vi "Toggle Debugging_Item_OnPopupMenu.vi"(11 "Object":T1) -> ()   [LabVIEW 2015]
uses:
  <resource>/Framework/Providers/API/ItemRef.ctl
  <resource>/Framework/Providers/API/mxLvMenuItem.ctl
panel:
  out "error out":errorcluster
  in  "error in":errorcluster
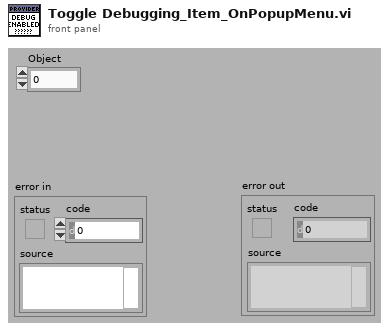
[diagram p1: front panel]
types:
  T1 = typedef "ItemRef.ctl" = u64
  T2 = typedef "mxLvMenuItem.ctl" = cluster{"Menu Name":string, "Description":string, "Icon File Name":path, "Menu Tag":string, "Enabled":bool, "Checked":bool, "Separator":bool, "Batchable":bool, "Weight":i32, "Batch Mode (Ignored if Not Batchable)":enum32{"Show If All Items Support Command", "Show If Any Items Support Command"}, "Menu Location":enum32{"<None>", "Project", "Project / Build Specifications", "Tools", "Tools / Source Control", "Tools / Real-Time Module", "Help"}, "Exclude From Getting Started Window Menu":bool}
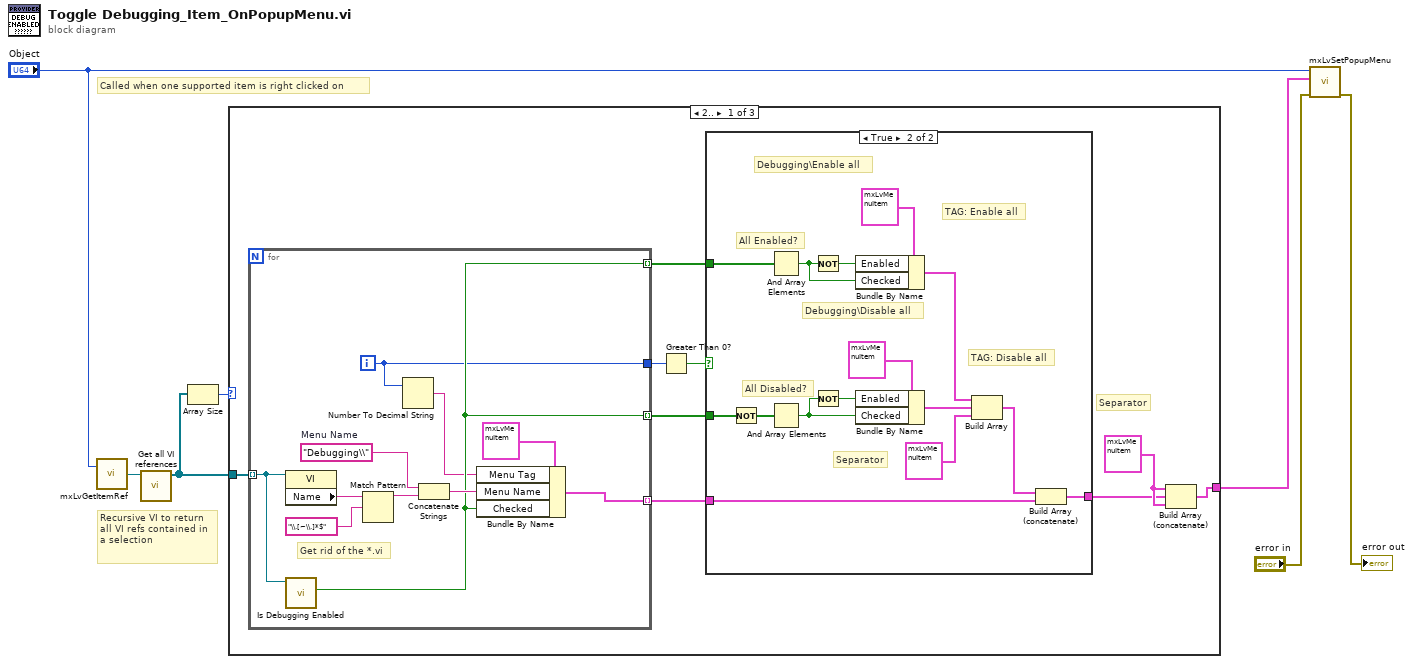
[diagram p0: block diagram]
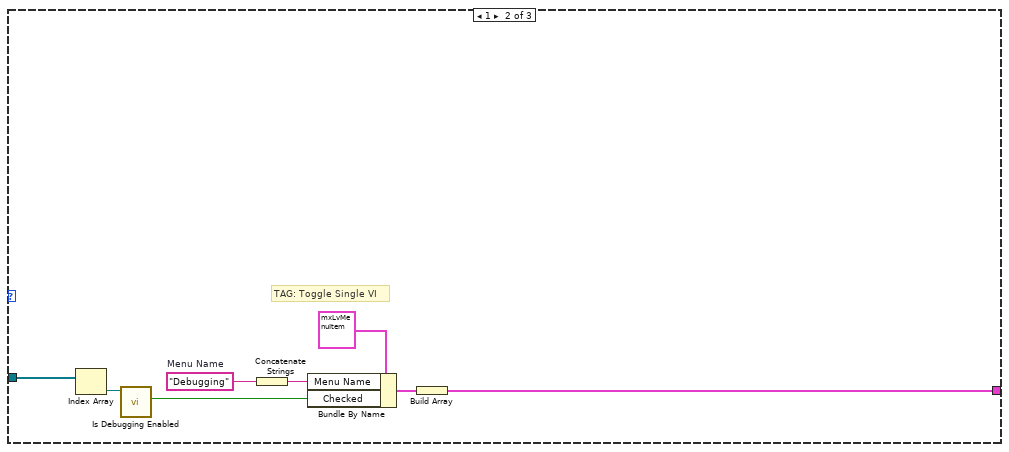
[diagram p3: hidden frame]
diagram:
  # "Recursive VI to return all VI refs contained in a selection"
  # "Called when one supported item is right clicked on"
  n1 = call <resource>:"mxLvGetItemRef.vi"("Item"="Object") -> ("Item Refnum"=w3:refnum<vi>)  [unwired: 1 in, 2 out]
  n2 = call "Get all VI references.vi"("Project Item"=w3) -> ("VI Refs"=w1:refnum<vi>[])  [unwired: 9 in, 1 out]
  n3 = Array Size(array=w1) -> (size(s)=w2:i32)
  n4 = case shown="2.." w2 {
    tunnel: [w15 w46 _] -> w4
    tunnel: w1 -> [w8 w45 _]
    frame 2.. {
      w16 = T2 {"Menu Name"="SEP", "Description"="", "Icon File Name"=path "", "Menu Tag"="SEP", "Enabled"=TRUE, "Checked"=FALSE, "Separator"=TRUE, "Batchable"=TRUE, "Weight"=0, "Batch Mode (Ignored if Not Batchable)"=enum."Show If All Items Support Command", "Menu Location"=enum."<None>", "Exclude From Getting Started Window Menu"=FALSE} ("Menu Item")
      # "Separator"
      # "Virtual Folder or Auto Populating Folder"
      n5 = for {
        tunnel: [w40] -> w12 mode=indexing
        tunnel: [w34] -> w10
        tunnel: [w38] -> w14 mode=indexing
        tunnel: [w38] -> w13 mode=indexing
        tunnel: w8 -> [w37] mode=indexing
        i -> [w34]
        w43 = "Debugging\\"  # Menu Name
        # "Get rid of the *.vi"
        n6 = property class="VI"(reference=w37) -> ("Name"=w36:string)  [unwired: 1 in, 2 out]
        n7 = call "Is Debugging Enabled.vi"("VI Reference In"=w37) -> ("Debugging Enabled?"=w38:bool)  [unwired: 8 in, 2 out]
        n8 = Match Pattern(string=w36, regular expression="\\.[~\\.]*$") -> (before substring=w35:string)  [unwired: 4 out]
        n9 = Number To Decimal String(number=w34) -> (decimal integer string=w33:string)  [unwired: 1 in]
        n10 = Concatenate Strings(w43, w35) -> (w41:string)
        n11 = Bundle By Name(cluster=T2 {"Menu Name"="", "Description"="", "Icon File Name"=path "", "Menu Tag"="Toggle Single VI", "Enabled"=TRUE, "Checked"=FALSE, "Separator"=FALSE, "Batchable"=TRUE, "Weight"=0, "Batch Mode (Ignored if Not Batchable)"=enum."Show If All Items Support Command", "Menu Location"=enum."<None>", "Exclude From Getting Started Window Menu"=FALSE} ("Menu Item"), "Menu Tag"=w33, "Menu Name"=w41, "Checked"=w38) -> (w40:T2)
      }
      n12 = Greater Than 0?(x=w10) -> (x > 0?=w9:bool)
      n13 = case shown="True" w9 {
        tunnel: w14 -> [_ w32]
        tunnel: w13 -> [_ w31]
        tunnel: w12 -> [w17 w19]
        tunnel: [w17 w18] -> w11
        frame False {
        }
        frame True {
          # "Debugging\\Enable all"
          # "TAG: Disable all"
          # "TAG: Enable all"
          # "Debugging\\Disable all"
          # "Separator"
          # "All Disabled?"
          # "All Enabled?"
          n14 = Not(x=w31) -> (.not. x?=w30:bool[])
          n15 = And Array Elements(Boolean array=w32) -> (logical AND=w28:bool)
          n16 = And Array Elements(Boolean array=w30) -> (logical AND=w24:bool)
          n17 = Not(x=w28) -> (.not. x?=w27:bool)
          n18 = Not(x=w24) -> (.not. x?=w25:bool)
          n19 = Bundle By Name(cluster=T2 {"Menu Name"="Debugging\\Enable all", "Description"="", "Icon File Name"=path "", "Menu Tag"="Enable all", "Enabled"=TRUE, "Checked"=FALSE, "Separator"=FALSE, "Batchable"=TRUE, "Weight"=0, "Batch Mode (Ignored if Not Batchable)"=enum."Show If All Items Support Command", "Menu Location"=enum."<None>", "Exclude From Getting Started Window Menu"=FALSE} ("Menu Item"), "Enabled"=w27, "Checked"=w28) -> (w23:T2)
          n20 = Bundle By Name(cluster=T2 {"Menu Name"="Debugging\\Disable all", "Description"="", "Icon File Name"=path "", "Menu Tag"="Disable all", "Enabled"=TRUE, "Checked"=FALSE, "Separator"=FALSE, "Batchable"=TRUE, "Weight"=0, "Batch Mode (Ignored if Not Batchable)"=enum."Show If All Items Support Command", "Menu Location"=enum."<None>", "Exclude From Getting Started Window Menu"=FALSE} ("Menu Item"), "Enabled"=w25, "Checked"=w24) -> (w22:T2)
          n21 = Build Array(w23, w22, T2 {"Menu Name"="Debugging\\SEP", "Description"="", "Icon File Name"=path "", "Menu Tag"="SEP", "Enabled"=TRUE, "Checked"=FALSE, "Separator"=TRUE, "Batchable"=TRUE, "Weight"=0, "Batch Mode (Ignored if Not Batchable)"=enum."Show If All Items Support Command", "Menu Location"=enum."<None>", "Exclude From Getting Started Window Menu"=FALSE} ("Menu Item")) -> (w20:T2[])
          n22 = Build Array (concatenate)(w20, w19) -> (w18:T2[])
        }
      }
      n23 = Build Array (concatenate)(w16, w11, w16) -> (w15:T2[])
    }
    frame 1 {
      w51 = "Debugging"  # Menu Name
      # "TAG: Toggle Single VI"
      n24 = Index Array(array=w45) -> (element=w44:refnum<vi>)  [unwired: 1 in]
      n25 = call "Is Debugging Enabled.vi"("VI Reference In"=w44) -> ("Debugging Enabled?"=w48:bool)  [unwired: 8 in, 2 out]
      n26 = Concatenate Strings(w51) -> (w49:string)
      n27 = Bundle By Name(cluster=T2 {"Menu Name"="", "Description"="", "Icon File Name"=path "", "Menu Tag"="Toggle Single VI", "Enabled"=TRUE, "Checked"=FALSE, "Separator"=FALSE, "Batchable"=TRUE, "Weight"=0, "Batch Mode (Ignored if Not Batchable)"=enum."Show If All Items Support Command", "Menu Location"=enum."<None>", "Exclude From Getting Started Window Menu"=FALSE} ("Menu Item"), "Menu Name"=w49, "Checked"=w48) -> (w47:T2)
      n28 = Build Array(w47) -> (w46:T2[])
    }
    frame 0, Default {
    }
  }
  n29 = call <resource>:"mxLvSetPopupMenu.vi"("error in"="error in", "Popup Menu Items"=w4, "Item"="Object") -> ("error out"=→"error out":errorcluster)  [unwired: 7 in, 1 out]
